vi "Set Return Values.vi"(8 "error in (no error)":errorcluster, 10 "VI Reference":refnum<vi>, 11 "Mock In":refnum<class "Mock.lvclass">) -> (3 "Mock Out":refnum<class "Mock.lvclass">)   [LabVIEW 2020, in "Mock.lvclass"]
uses:
  Mock.lvclass
  Mock.lvclass/Mock.ctl
  VI Call/VI Call.lvclass
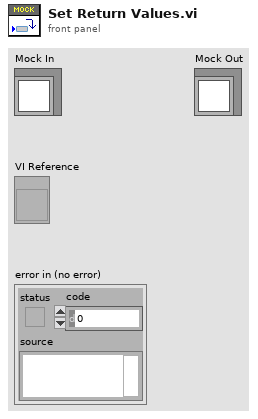
[diagram p1: front panel]
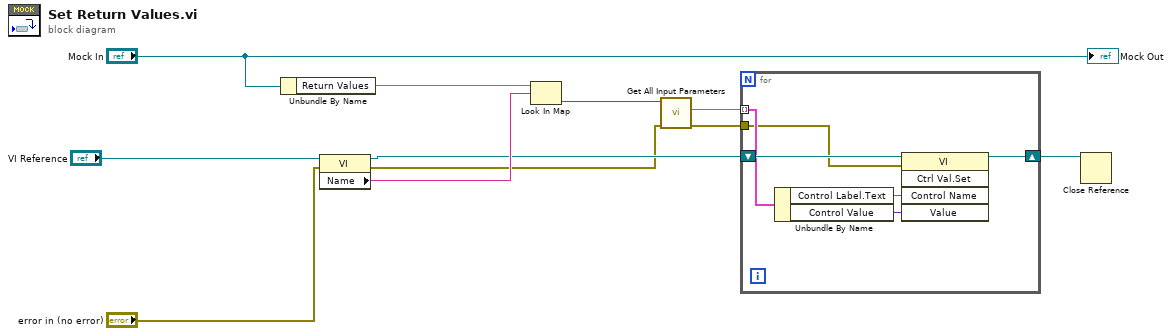
[diagram p0: block diagram]
diagram:
  n1 = Unbundle By Name("Mock In") -> ("Return Values"=w9:map{string, refnum<class "VI Call.lvclass">})
  n2 = property class="VI"(reference="VI Reference", error in="error in (no error)") -> (reference out=w6:refnum<vi>, error out=w4:errorcluster, "Name"=w8:string)
  n3 = Look In Map(map=w9, key=w8) -> (value=w7:refnum<class "VI Call.lvclass">)  [unwired: 1 in, 1 out]
  n4 = call-dynamic "Get All Input Parameters.vi"("error in (no error)"=w4, "VI Call In"=w7) -> ("error out"=w1:errorcluster, "Input Parameters"=w5:map{string, variant})  [unwired: 8 in]
  n5 = for {
    tunnel: w5 -> [w16] mode=indexing
    shift-right: [w13] -> w2
    shift-left: w6 -> [w17]
    tunnel: w1 -> [w12]
    n6 = Unbundle By Name(w16) -> ("Control Label.Text"=w14:string, "Control Value"=w15:variant)
    n7 = invoke class="VI" method="Ctrl Val.Set"(reference=w17, error in=w12, "Control Name"=w14, "Value"=w15) -> (reference out=w13:refnum<vi>)  [unwired: 1 in, 4 out]
  }
  n8 = Close Reference(reference=w2) -> ()  [unwired: 1 in, 1 out]
  "Mock Out" <- "Mock In"
